vi "Plot 2 data.vi"() -> ()   [LabVIEW 2019]
panel:
  in  "stop":bool
  out "Waveform Graph":cluster{dbl, dbl, dbl[][]}(graph)
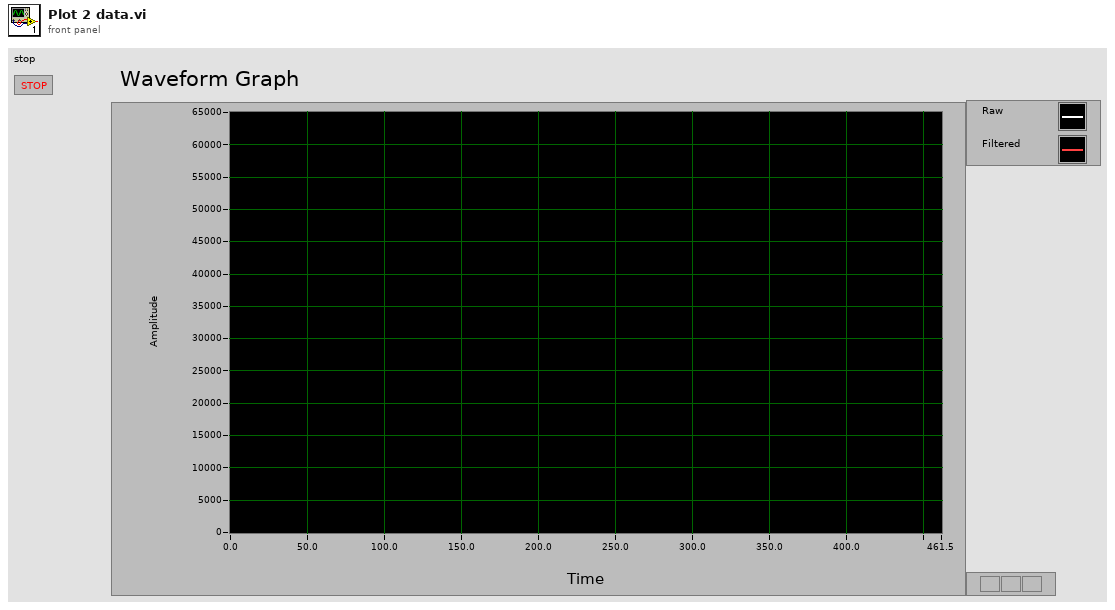
[diagram p1: front panel]
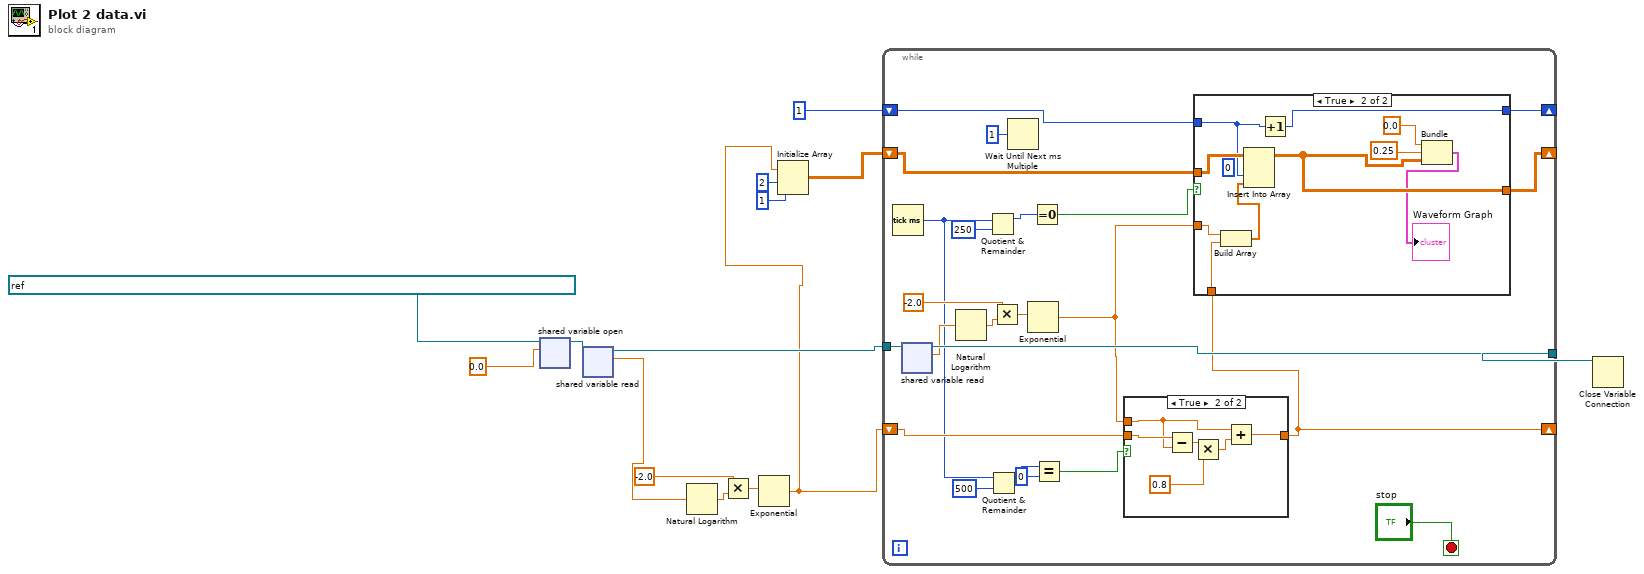
[diagram p0: block diagram]
diagram:
  n1 = shared-variable-open(refnum<k21> "ni.var.psp://huniopc01/NiCorpOPC_IO/NIOPCCorp/TDK Sputter/PLC/Vacuum/Main_Chmbr_CM_Targ" ("shared variable refnum in"), 0.0) -> (w11:refnum<k21>)  [unwired: 2 in, 1 out]
  n2 = shared-variable-read(w11) -> (w10:refnum<k21>, w6:dbl)  [unwired: 1 in, 2 out]
  n3 = Natural Logarithm(1:w6) -> (0:w9:dbl)
  n4 = Multiply(x=-2.0, y=w9) -> (x*y=w7:dbl)
  n5 = Exponential(1:w7) -> (0:w4:dbl)
  n6 = Initialize Array(w4, 2 ("dimension size"), 1 ("dimension size")) -> (w3:dbl[][])
  n7 = while {
    tunnel: w10 -> [w37]
    tunnel: [w36] -> w13
    shift-right: [w28] -> _
    shift-left: w4 -> [w29]
    shift-right: [w17] -> _
    shift-left: w3 -> [w18]
    shift-right: [w15] -> _
    shift-left: 1 -> [w16]
    stop <- "stop" stop-if-true
    n8 = Tick Count (ms)() -> (millisecond timer value=w19:u32)
    n9 = shared-variable-read(w37) -> (w36:refnum<k21>, w27:dbl)  [unwired: 1 in, 2 out]
    n10 = Natural Logarithm(1:w27) -> (0:w26:dbl)
    n11 = Quotient & Remainder(x=w19, y=u32 250) -> (x-y*floor(x/y)=w21:u32)  [unwired: 1 out]
    n12 = Quotient & Remainder(x=w19, y=500) -> (x-y*floor(x/y)=w32:u32)  [unwired: 1 out]
    n13 = Multiply(x=-2.0, y=w26) -> (x*y=w24:dbl)
    n14 = Wait Until Next ms Multiple(millisecond multiple=u32 1) -> ()  [unwired: 1 out]
    n15 = Exponential(1:w24) -> (0:w23:dbl)
    n16 = Equal To 0?(x=w21) -> (x = 0?=w20:bool)
    n17 = Equal?(x=w32, y=0) -> (x = y?=w30:bool)
    n18 = case shown="True" w30 {
      tunnel: w23 -> [_ w51]
      tunnel: w29 -> [w50 w56]
      tunnel: [w50 w55] -> w28
      frame False {
      }
      frame True {
        n19 = Subtract(x=w56, y=w51) -> (x-y=w54:dbl)
        n20 = Multiply(x=w54, y=0.8) -> (x*y=w52:dbl)
        n21 = Add(x=w51, y=w52) -> (x+y=w55:dbl)
      }
    }
    n22 = case shown="True" w20 {
      tunnel: w28 -> [_ w47]
      tunnel: w23 -> [_ w45]
      tunnel: w18 -> [w39 w46]
      tunnel: [w39 w43] -> w17
      tunnel: w16 -> [w38 w42]
      tunnel: [w38 w41] -> w15
      frame False {
      }
      frame True {
        (unwired) 0 ("index (row)")
        n23 = Build Array(w45, w47) -> (w44:dbl[])
        n24 = Insert Into Array(array=w46, index (col)=w42, new element=w44) -> (w43:dbl[][])  [unwired: 1 in]
        n25 = Increment(x=w42) -> (x+1=w41:i32)
        n26 = Bundle(0.0, 0.25, w43) -> (→"Waveform Graph":cluster{dbl, dbl, dbl[][]})  [unwired: 1 in]
      }
    }
  }
  n27 = Close Variable Connection(11:w13) -> ()  [unwired: 1 in, 1 out]
